vi "TDMS_Write_Channel_Schedule.vi"(8 "error in (no error)":errorcluster, 10 "output cluster":T1, 11 "Refnum in":refnum<k34>) -> (0 "error out":errorcluster)   [LabVIEW 2016]
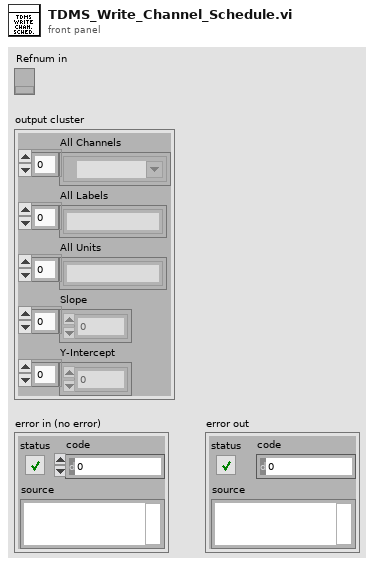
[diagram p1: front panel]
types:
  T1 = cluster{"All Channels":tag[], "All Labels":string[], "All Units":string[], "Slope":dbl[], "Y-Intercept":dbl[]}
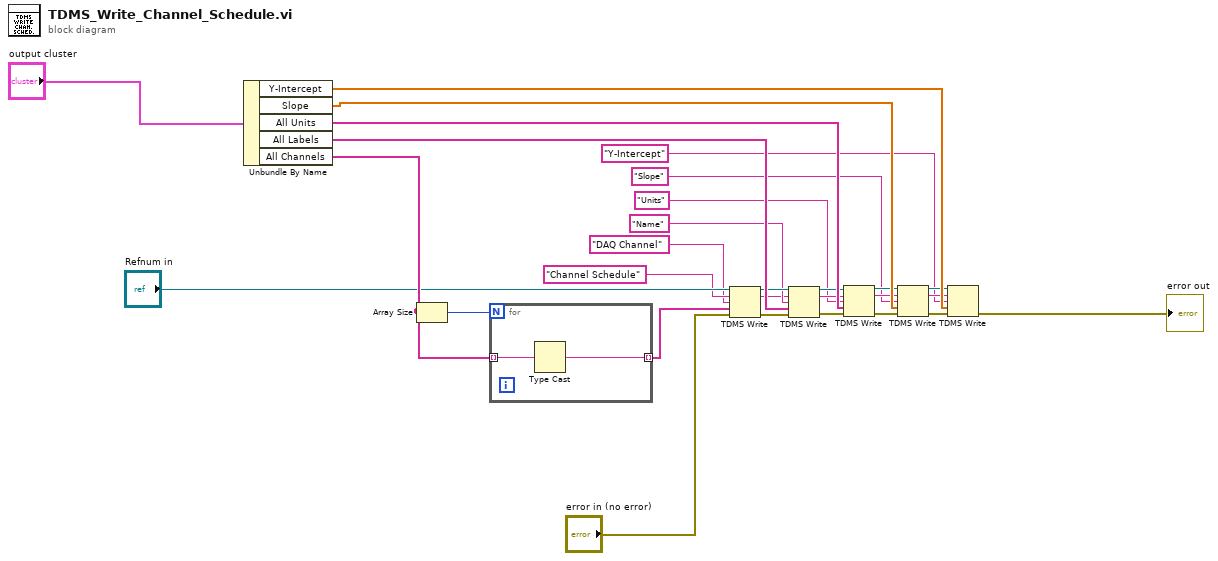
[diagram p0: block diagram]
diagram:
  n1 = Unbundle By Name("output cluster") -> ("Y-Intercept"=w29:dbl[], "Slope"=w28:dbl[], "All Units"=w27:string[], "All Labels"=w26:string[], "All Channels"=w25:tag[])
  n2 = Array Size(array=w25) -> (size(s)=w22:i32)
  n3 = for {
    N: w22 -> [_]
    tunnel: w25 -> [w31] mode=indexing
    tunnel: [w30] -> w21 mode=indexing
    n4 = Type Cast(x=w31) -> (*(type *) &x=w30:string)  [unwired: 1 in]
  }
  n5 = TDMS Write(0:"Refnum in", 5:"Channel Schedule" ("channel name(s) in (Untitled)"), 7:"DAQ Channel" ("group name in (Untitled)"), 9:w21, 11:"error in (no error)") -> (4:w20:refnum<k34>, 6:w12:string, 15:w14:errorcluster)  [unwired: 1 in, 1 out]
  n6 = TDMS Write(0:w20, 5:w12, 7:"Name" ("group name in (Untitled)"), 9:w26, 11:w14) -> (4:w19:refnum<k34>, 6:w11:string, 15:w15:errorcluster)  [unwired: 1 in, 1 out]
  n7 = TDMS Write(0:w19, 5:w11, 7:"Units" ("group name in (Untitled)"), 9:w27, 11:w15) -> (4:w18:refnum<k34>, 6:w10:string, 15:w16:errorcluster)  [unwired: 1 in, 1 out]
  n8 = TDMS Write(0:w18, 5:w10, 7:"Slope" ("group name in (Untitled)"), 9:w28, 11:w16) -> (4:w8:refnum<k34>, 6:w9:string, 15:w17:errorcluster)  [unwired: 1 in, 1 out]
  n9 = TDMS Write(0:w8, 5:w9, 7:"Y-Intercept" ("group name in (Untitled)"), 9:w29, 11:w17) -> (15:→"error out":errorcluster)  [unwired: 1 in, 3 out]
